vi "TCP Write Bytes.vi"(8 "error in (no error)":errorcluster, 9 "timeout ms (2000)":i32=2000, 10 "Bytes":u8[](array[numeric]) format="%08b", 11 "Connection.TCP":refnum<class "Connection.TCP.lvclass">) -> (0 "error out":errorcluster, 3 "Connection.TCP":refnum<class "Connection.TCP.lvclass">)   [LabVIEW 2013, in "Connection.TCP_GOSPL.lvlib" / "Connection.TCP.lvclass"]
uses:
  Connection.TCP.lvclass
  Connection.TCP.lvclass/Connection.TCP.ctl
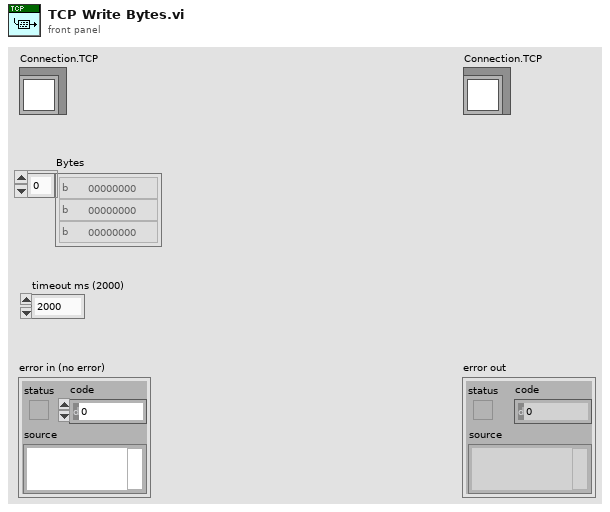
[diagram p1: front panel]
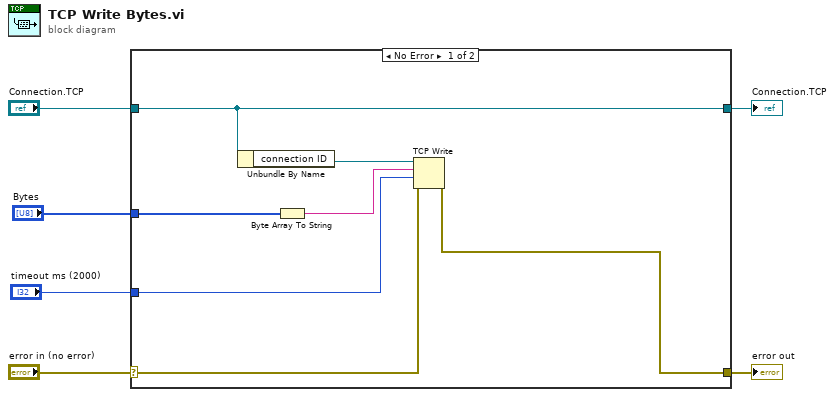
[diagram p0: block diagram]
diagram:
  n1 = case shown="No Error" "error in (no error)" {
    selector: "error in (no error)" -> [w9 w15]
    tunnel: [w8 w15] -> w5
    tunnel: [w13 w14] -> w3
    tunnel: "Connection.TCP" -> [w13 w14]
    tunnel: "Bytes" -> [w11 _]
    tunnel: "timeout ms (2000)" -> [w7 _]
    frame No Error {
      n2 = Unbundle By Name(w13) -> ("connection ID"=w12:refnum<k5>)
      n3 = Byte Array To String(unsigned byte array=w11) -> (string=w10:string)
      n4 = TCP Write(connection ID=w12, data in=w10, error in (no error)=w9, 9:w7) -> (error out=w8:errorcluster)  [unwired: 2 out]
    }
    frame Error {
    }
  }
  "error out" <- w5
  "Connection.TCP" <- w3
